vi "Open Websocket Connection.vi"(4 "timeout hand shake [ms]":i32, 6 "WS Server Port":string, 7 "timeout opening [ms]":i32, 8 "error in (no error)":errorcluster, 9 "Connection Retries":i32=7, 10 "WS Server IP":string, 11 "Data Cluster in":T1) -> (0 "error out":errorcluster, 2 "Return Headers":variant, 3 "Data Cluster out":T1)   [LabVIEW 2020, in "horiba.lvlib" / "DeviceManager.lvlib"]
doc: "This VI implements local error handling for opening the websocket connection:\nThe ICL first looks if it is licensed and after that is open for websocket connections. \nSo it the underlaying TCP connection errors out, this VI waits for 2 seconds and tries up to 5 times to establish the connection. After that it errors out."
uses:
  DeviceManager.lvlib
  ICLcommuncationData.ctl
  Communicator/Communicator.lvclass
  719029ff-c35a-4930-a5c1-7c3d91bcc3d6.vi
  <vilib>/GPower/Error/Library/ErrorType.vi
  <vilib>/GPower/Error/Library/SplitAppended.vi
  <vilib>/Utility/error.llb/Trim Whitespace.vi
  <vilib>/GPower/Error/Library/SubVIs/ExplanationToError.vi
  <vilib>/Utility/error.llb/Trim Whitespace One-Sided.vi
  <vilib>/dlg_ctls.llb/Space Constant.vi
  <vilib>/Utility/error.llb/Error Code Database.vi
  <vilib>/GPower/Error/Library/SubVIs/SetStatus.vi
  <vilib>/GPower/Error/Library/AppendErrors.vi
  <vilib>/GPower/Error/Library/Append/AppendSingle.vi
  <vilib>/GPower/Error/GPError.lvlib
  <vilib>/Hampel Software Engineering/HSE Logger/hse-logger.lvlib
panel:
  # "Connector Pane"
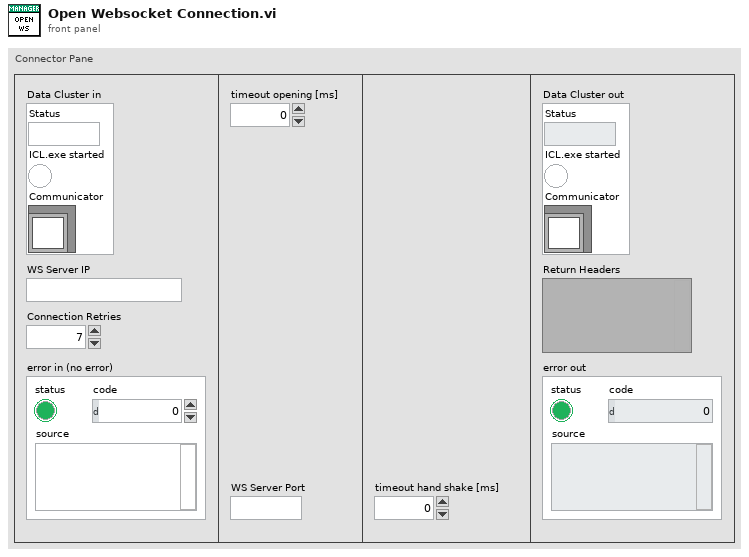
[diagram p1: front panel]
types:
  T1 = typedef "horiba.lvlib/DeviceManager.lvlib/ICLcommuncationData.ctl" = cluster{"Status":string, "ICL.exe started":bool, "Communicator":refnum<class "Communicator.lvclass">}
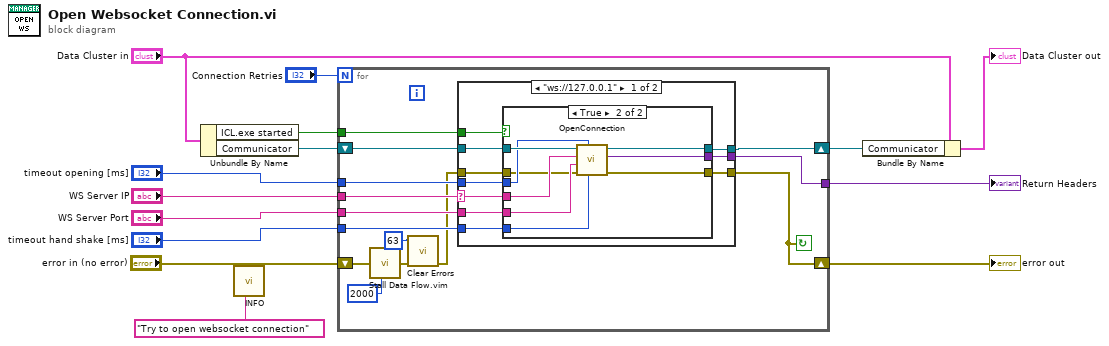
[diagram p0: block diagram]
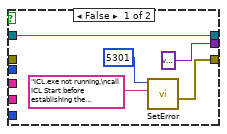
[diagram p2: hidden frame]
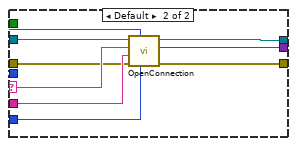
[diagram p3: hidden frame]
diagram:
  n1 = Unbundle By Name("Data Cluster in") -> ("ICL.exe started"=w4:bool, "Communicator"=w5:refnum<class "Communicator.lvclass">)
  n2 = call <vilib>:"INFO.vi"("Message"="Try to open websocket connection") -> ()  [unwired: 10 in, 1 out]
  n3 = for {
    N: "Connection Retries" -> [_]
    tunnel: "WS Server IP" -> [w28]
    tunnel: "timeout opening [ms]" -> [w25]
    tunnel: "timeout hand shake [ms]" -> [w24]
    tunnel: "WS Server Port" -> [w23]
    tunnel: w4 -> [w21]
    tunnel: [w20] -> w3
    shift-right: [w15] -> w12
    shift-left: "error in (no error)" -> [w27]
    shift-right: [w26] -> w11
    shift-left: w5 -> [w22]
    stop <- w15 continue-if-true
    n4 = call "Stall Data Flow.vim"("value in"=w27, "milliseconds to wait"=u32 2000) -> ("value out"=w19:errorcluster)  [unwired: 1 out]
    n5 = call <vilib>:"Clear Errors.vi"("error in (no error)"=w19, "specific error code to clear (0: all)"=63) -> ("error out"=w17:errorcluster)  [unwired: 4 in, 1 out]
    n6 = case shown="\"ws://127.0.0.1\"" w28 {
      selector: w28 -> [w35 w59]
      tunnel: w21 -> [w38 _]
      tunnel: w22 -> [w37 w61]
      tunnel: w23 -> [w36 w60]
      tunnel: w24 -> [w34 w58]
      tunnel: w25 -> [w33 w57]
      tunnel: [w32 w56] -> w26
      tunnel: [w31 w55] -> w15
      tunnel: w17 -> [w30 w54]
      tunnel: [w29 w53] -> w20
      frame "ws://127.0.0.1" {
        n7 = case shown="True" w38 {
          tunnel: [w41 w47] -> w31
          tunnel: [variant ("Return Headers") w46] -> w29
          tunnel: w37 -> [w39 w52]
          tunnel: w36 -> [_ w51]
          tunnel: w35 -> [_ w50]
          tunnel: w34 -> [_ w49]
          tunnel: w33 -> [_ w48]
          tunnel: [w39 w45] -> w32
          tunnel: w30 -> [_ w44]
          frame False {
            n8 = call <vilib>:"SetError.vi"("Error description"="ICL.exe not running,\ncall ICL Start before establishing the communication", "Error code"=5301) -> ("Error out"=w41:errorcluster)  [unwired: 9 in]
          }
          frame True {
            n9 = call-dynamic "OpenConnection.vi"("timeout hand shake [ms]"=w49, "timeout opening [ms]"=w48, "error in (no error)"=w44, "WS Server Port"=w51, "WS Server IP"=w50, "Communicator in"=w52) -> ("error out"=w47:errorcluster, "Return Headers"=w46:variant, "Communicator out"=w45:refnum<class "Communicator.lvclass">)  [unwired: 3 in]
          }
        }
      }
      frame Default {
        n10 = call-dynamic "OpenConnection.vi"("timeout hand shake [ms]"=w58, "timeout opening [ms]"=w57, "error in (no error)"=w54, "WS Server Port"=w60, "WS Server IP"=w59, "Communicator in"=w61) -> ("error out"=w55:errorcluster, "Return Headers"=w53:variant, "Communicator out"=w56:refnum<class "Communicator.lvclass">)  [unwired: 3 in]
      }
    }
  }
  "error out" <- w12
  "Return Headers" <- w3
  n11 = Bundle By Name(cluster="Data Cluster in", "Communicator"=w11) -> (→"Data Cluster out":T1)
